vi "SENS_CORR_CSET_GUID_S.vi"(0 "VISA IN":refnum<visa-resource-name>, 1 "Calset GUID":string, 5 "error in":errorcluster, 7 "Channel":i32) -> (14 "VISA Out":refnum<visa-resource-name>, 19 "error out":errorcluster)   [LabVIEW 2018, in "PNA-X.lvlib"]
doc: "SENSe<cnum>:CORRection:CSET:GUID <string> Superseded \n1694\n\nThis command is replaced by SENS:CORR:CSET:ACTivate. \n(Read-Write) Selects the Cal Set identified by the string parameter (GUID) and applies it to the \nspecified channel. \nA Cal Set cannot be selected for a channel which is not ON. \nIf the stimulus settings of the selected Cal Set differ from those of the selected channel, the instrument will \nautomatically change the channel's settings to match the Cal Set. \nParameters \n<cnum> Any existing channel number. If unspecified, value is set to 1 \n<string> GUID of the desired Cal Set. The curly brackets and hyphens must be included. \nExamples SENS:CORR:CSET:GUID '{2B893E7A-971A-11d5-8D6C-00108334AE96}' \nsense2:correction:cset:guid '{2B893E7A-971A-11d5-8D6C- \n00108334AE96}' \nQuery Syntax SENSe<cnum>:CORRection:CSET:GUID? \nReturns the GUID of the currently-selected Cal Set for the specified \nchannel. \nReturn Type String \nDefault Not Applicable"
uses:
  PNA-X.lvlib
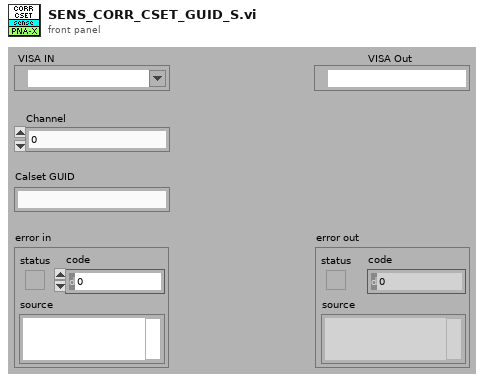
[diagram p1: front panel]
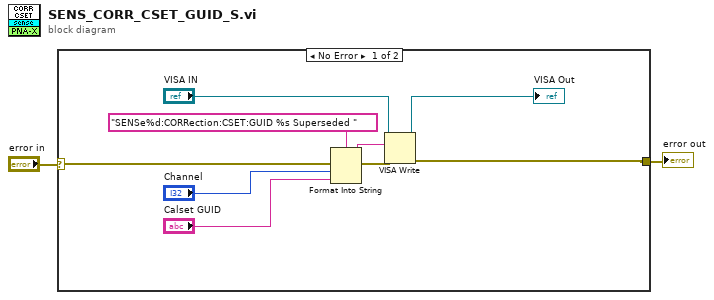
[diagram p0: block diagram]
diagram:
  n1 = case shown="No Error" "error in" {
    selector: "error in" -> [w11 w12]
    tunnel: [w6 w12] -> w1
    frame No Error {
      n2 = Format Into String(format string="SENSe%d:CORRection:CSET:GUID %s Superseded " ("Cmdline"), error in=w11, "Channel", "Calset GUID") -> (resulting string=w9:string, error out=w10:errorcluster)  [unwired: 1 in]
      n3 = VISA Write(VISA resource name="VISA IN", write buffer=w9, error in (no error)=w10) -> (VISA resource name out=→"VISA Out":refnum<visa-resource-name>, error out=w6:errorcluster)  [unwired: 1 out]
    }
    frame Error {
    }
  }
  "error out" <- w1
